vi "Battery.vi"() -> ()   [LabVIEW 2018]
uses:
  <vilib>/OPCUA/controls/NodeIds.ctl
  <vilib>/OPCUA/controls/NodeId.ctl
  GlobalVal.vi
  <vilib>/OPCUA/client/Multiple Read Variant.vi
  <vilib>/OPCUA/NI OPC UA Client.lvlib
panel:
  in  "BT001_Ki":dbl
  in  "BT001_Kp":dbl
  in  "BT001_tp":dbl
  in  "BT001_kP":dbl
  in  "BT001_tf":dbl
  in  "BT001_kf":dbl
  out "BT001_tf":dbl
  out "DS001_Ki":dbl
  out "BT001_tP":dbl caption="DS001_tP"
  out "BT001_kf":dbl caption="DS001_kf"
  out "BT001_kP":dbl caption="DS001_kP"
  out "BT001_Kp":dbl caption="DS001_Kp"
  out "BT001_Thermo":dbl(slide) scale=0.0..100.0
  out "BT001_SOC":dbl(knob) scale=0.0..100.0
  out "OPCUA Error Log":errorcluster
  out "OPC Server URL":string
  out "BT001_f0, f Chart":cluster{dbl, dbl}(graph)
  out "BT001_P0, P Chart":cluster{dbl, dbl}(graph)
  out "Time Stamp":timestamp
  out "Pmin":dbl(slide) scale=480.0..510.0
  out "Pmax":dbl(slide) scale=10.0..60.0
  in  "stop":bool
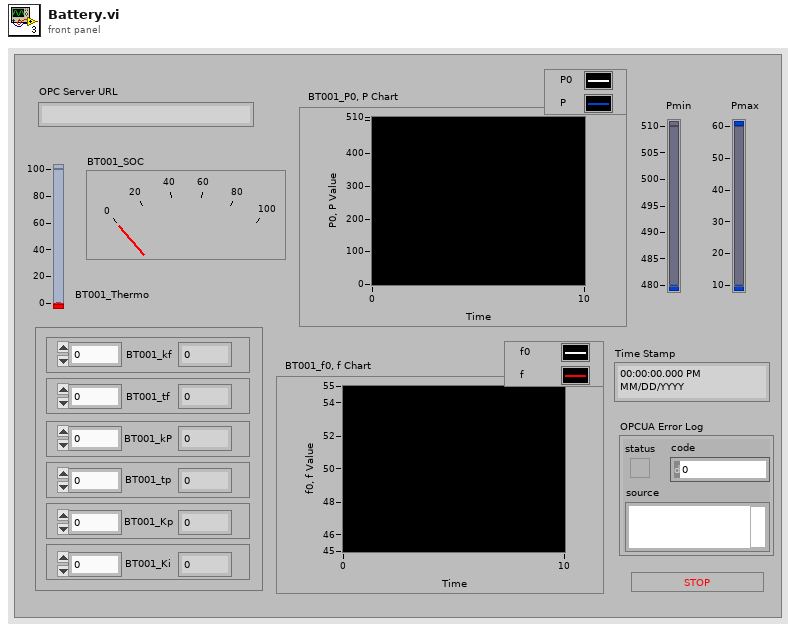
[diagram p1: front panel]
types:
  T1 = typedef "OPC UA Client Refnum.ctl" = refnum<k21>
  T2 = typedef "NodeIds.ctl" = T3[]
  T3 = typedef "NodeId.ctl" = string
  T4 = typedef "Read Variant Result.ctl" = cluster{"node ID":T3, "value ":variant, "timestamp":timestamp, "status":T5}
  T5 = typedef "OPC UA StatusCode.ctl" = u32
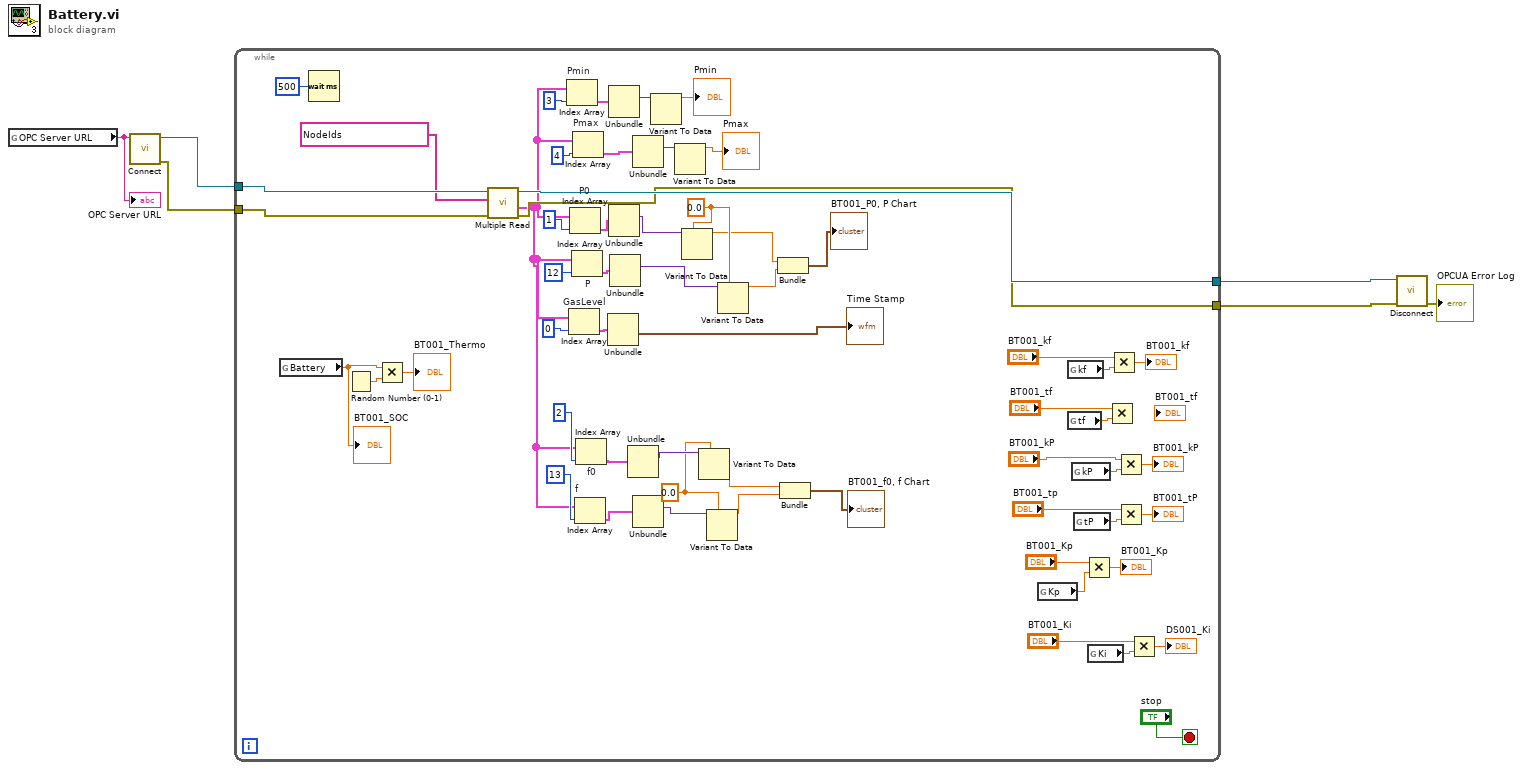
[diagram p0: block diagram]
diagram:
  n1 = global read "GlobalVal.vi" "OPC Server URL"() -> (w1:string)
  "OPC Server URL" <- w1
  n2 = call <vilib>:"Connect.vi"("server endpoint URL"=w1) -> ("error out"=w5:errorcluster, "OPC UA client refnum out"=w6:T1)  [unwired: 8 in, 1 out]
  n3 = while {
    tunnel: w6 -> [w64]
    tunnel: w5 -> [w63]
    tunnel: [w61] -> w4
    tunnel: [w60] -> w3
    stop <- "stop" stop-if-true
    w31 = 0.0
    w41 = 0.0
    n4 = global read "GlobalVal.vi" "Battery"() -> (w26:dbl)
    "BT001_SOC" <- w26
    n5 = Wait (ms)(milliseconds to wait=u32 500) -> ()  [unwired: 1 out]
    n6 = Random Number (0-1)() -> (number: 0 to 1=w24:dbl)
    n7 = Multiply(x=w26, y=w24) -> (x*y=→"BT001_Thermo":dbl)
    n8 = call-poly <vilib>:"Multiple Read.vi"("error in (no error)"=w63, "node IDs"=T2 ["ns=2;i=2", "ns=2;i=3", "ns=2;i=4", "ns=2;i=5", "ns=2;i=6", "ns=2;i=7", "ns=2;i=8", "ns=2;i=9", "ns=2;i=10", "ns=2;i=11", "ns=2;i=12", "ns=2;i=13", "ns=2;i=14", "ns=2;i=15"], "OPC UA client refnum in"=w64) -> ("error out"=w60:errorcluster, "results"=w27:T4[], "OPC UA client refnum out"=w61:T1)  [unwired: 5 in, 1 out]
    n9 = Index Array "Pmin"(array=w27, index=3) -> (element=w53:T4)
    n10 = Index Array "GasLevel"(array=w27, index=0) -> (element=w57:T4)
    n11 = Index Array "P0"(array=w27, index=1) -> (element=w55:T4)
    n12 = Index Array "P"(array=w27, index=12) -> (element=w44:T4)
    n13 = Index Array "Pmax"(array=w27, index=4) -> (element=w49:T4)
    n14 = Index Array "f"(array=w27, index=13) -> (element=w33:T4)
    n15 = Index Array "f0"(array=w27, index=2) -> (element=w36:T4)
    n16 = Unbundle(w57) -> ("timestamp"=→"Time Stamp":timestamp)  [unwired: 3 out]
    n17 = Unbundle(w53) -> ("value"=w52:variant)  [unwired: 3 out]
    n18 = Unbundle(w55) -> ("value"=w43:variant)  [unwired: 3 out]
    n19 = Unbundle(w44) -> ("value"=w42:variant)  [unwired: 3 out]
    n20 = Unbundle(w36) -> ("value"=w35:variant)  [unwired: 3 out]
    n21 = Unbundle(w49) -> ("value"=w48:variant)  [unwired: 3 out]
    n22 = Unbundle(w33) -> ("value"=w32:variant)  [unwired: 3 out]
    n23 = Variant To Data(Variant=w52) -> (data=→"Pmin":dbl)  [unwired: 2 in, 1 out]
    n24 = Variant To Data(Variant=w48) -> (data=→"Pmax":dbl)  [unwired: 2 in, 1 out]
    n25 = Variant To Data(type=w41, Variant=w43) -> (data=w38:dbl)  [unwired: 1 in, 1 out]
    n26 = Variant To Data(type=w31, Variant=w35) -> (data=w30:dbl)  [unwired: 1 in, 1 out]
    n27 = Variant To Data(type=w31, Variant=w32) -> (data=w29:dbl)  [unwired: 1 in, 1 out]
    n28 = Variant To Data(type=w41, Variant=w42) -> (data=w39:dbl)  [unwired: 1 in, 1 out]
    n29 = Bundle(w38, w39) -> (→"BT001_P0, P Chart":cluster{dbl, dbl})  [unwired: 1 in]
    n30 = Bundle(w30, w29) -> (→"BT001_f0, f Chart":cluster{dbl, dbl})  [unwired: 1 in]
    n31 = global read "GlobalVal.vi" "Kp"() -> (w10:dbl)
    n32 = global read "GlobalVal.vi" "kf"() -> (w21:dbl)
    n33 = global read "GlobalVal.vi" "tf"() -> (w19:dbl)
    n34 = global read "GlobalVal.vi" "kP"() -> (w16:dbl)
    n35 = global read "GlobalVal.vi" "tP"() -> (w14:dbl)
    n36 = Multiply(x="BT001_Kp", y=w10) -> (x*y=→"BT001_Kp":dbl)
    n37 = global read "GlobalVal.vi" "Ki"() -> (w7:dbl)
    n38 = Multiply(x="BT001_tf", y=w19) -> ()  [unwired: 1 out]
    n39 = Multiply(x="BT001_kf", y=w21) -> (x*y=→"BT001_kf":dbl)
    n40 = Multiply(x="BT001_kP", y=w16) -> (x*y=→"BT001_kP":dbl)
    n41 = Multiply(x="BT001_tp", y=w14) -> (x*y=→"BT001_tP":dbl)
    n42 = Multiply(x="BT001_Ki", y=w7) -> (x*y=→"DS001_Ki":dbl)
  }
  n43 = call <vilib>:"Disconnect.vi"("error in (no error)"=w3, "OPC UA client refnum in"=w4) -> ("error out"=→"OPCUA Error Log":errorcluster)  [unwired: 9 in]
